vi "MASTERSLAVE.vi"(8 "error in (no error)":errorcluster, 10 "Arg":string, 11 "Tapedrive_ESP301 in":refnum<class "Tapedrive_ESP301.lvclass">) -> (0 "error out":errorcluster, 3 "Tapedrive_ESP301 out":refnum<class "Tapedrive_ESP301.lvclass">)   [LabVIEW 2013, in "Tapedrive_ESP301.lvclass"]
uses:
  Tapedrive_ESP301.lvclass
  Direction.ctl
  shared/CompressAndUpdate(Poly)/CompressAndUpdate(Enum).vi
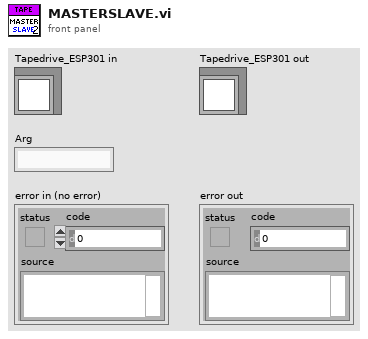
[diagram p1: front panel]
types:
  T1 = typedef "Direction.ctl" = enum16{"Forward", "Backward", "Undefined"}
  T2 = enum16{"Trapezoidal Mode", "S-curve Mode", "Jog Mode", "Slave to master's desired position (trajectory)", "Slave to master's actual position (feedback)", "Slave to master's actual velocity for jogging"}
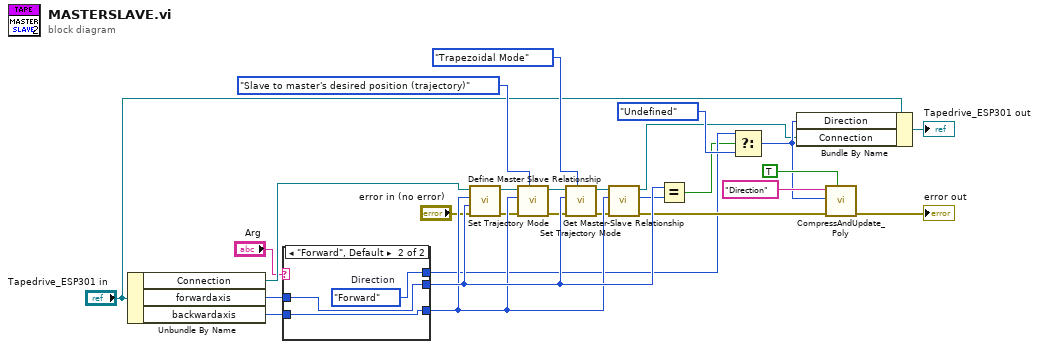
[diagram p0: block diagram]
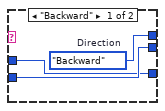
[diagram p2: hidden frame]
diagram:
  n1 = Unbundle By Name("Tapedrive_ESP301 in") -> ("Connection"=w8:refnum<visa-resource-name>, "forwardaxis"=w6:i16, "backwardaxis"=w7:i16)
  n2 = case shown="\"Forward\", Default" "Arg" {
    tunnel: w6 -> [w29 w33]
    tunnel: w7 -> [w30 w32]
    tunnel: [w30 w33] -> w27
    tunnel: [w29 w32] -> w26
    tunnel: [w28 w31] -> w19
    frame "Backward" {
      w28 = Direction."Backward"  # Direction
    }
    frame "Forward", Default {
      w31 = Direction."Forward"  # Direction
    }
  }
  n3 = call <instrlib>:"Define Master Slave Relationship.vi"("error in (no error)"="error in (no error)", "Master Axis"=w27, "Slave Axis"=w26, "VISA resource name"=w8) -> ("error out"=w4:errorcluster, "VISA resource name out"=w5:refnum<visa-resource-name>)  [unwired: 2 in]
  n4 = call <instrlib>:"Set Trajectory Mode.vi"("Trajectory Mode"=T2."Slave to master's desired position (trajectory)", "error in (no error)"=w4, "Axis (1)"=w26, "VISA resource name"=w5) -> ("error out"=w2:errorcluster, "VISA resource name out"=w3:refnum<visa-resource-name>)  [unwired: 3 in]
  n5 = call <instrlib>:"Set Trajectory Mode.vi"("Trajectory Mode"=T2."Trapezoidal Mode", "error in (no error)"=w2, "Axis (1)"=w27, "VISA resource name"=w3) -> ("error out"=w12:errorcluster, "VISA resource name out"=w14:refnum<visa-resource-name>)  [unwired: 3 in]
  n6 = call <instrlib>:"Get Master-Slave Relationship.vi"("error in (no error)"=w12, "Slave Axis"=w26, "VISA resource name"=w14) -> ("error out"=w22:errorcluster, "Master Axis"=w17:i32, "VISA resource name out"=w13:refnum<visa-resource-name>)  [unwired: 2 in]
  n7 = Equal?(x=w27, y=w17) -> (x = y?=w18:bool)
  n8 = Select(t=w19, s=w18, f=Direction."Undefined") -> (s? t:f=w21:T1)
  n9 = Bundle By Name(cluster="Tapedrive_ESP301 in", "Direction"=w21, "Connection"=w13) -> (→"Tapedrive_ESP301 out":refnum<class "Tapedrive_ESP301.lvclass">)
  n10 = call-poly "CompressAndUpdate_Poly.vi"("force CVT update (false)"=TRUE, "error in"=w22, "enum variant"=w21, "command or variable name"="Direction") -> ("error out"=→"error out":errorcluster)  [unwired: 7 in]
